vi "RGB to HSL.vi"(8 "error in (no error)":errorcluster, 9 "Blue":u8, 10 "Green":u8, 11 "Red":u8) -> (0 "error out":errorcluster, 1 "Lightness(%)":dbl format="%#_13g", 2 "Saturation(%)":dbl format="%#_13g", 3 "Hue(°)":dbl format="%#_13g")   [LabVIEW 2018]
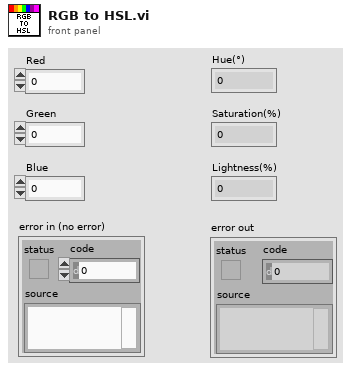
[diagram p1: front panel]
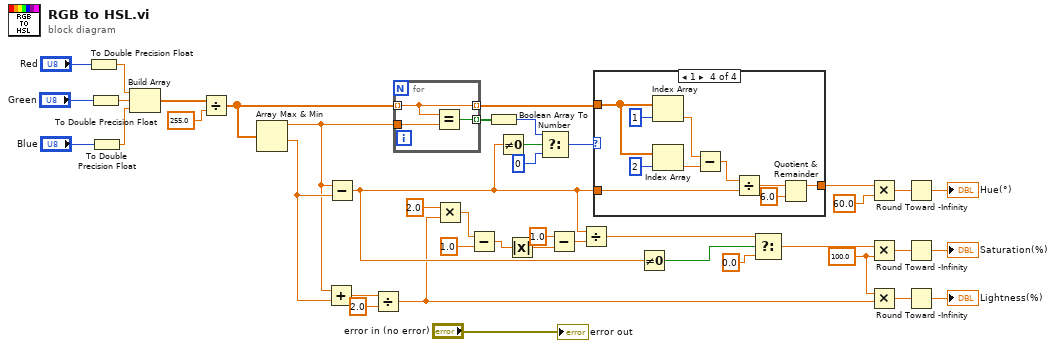
[diagram p0: block diagram]
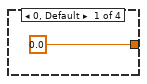
[diagram p2: hidden frame]
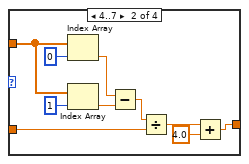
[diagram p3: hidden frame]
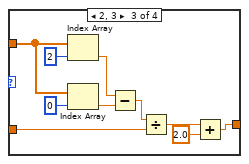
[diagram p4: hidden frame]
diagram:
  w31 = 100.0 ("x")
  n1 = To Double Precision Float(number="Red") -> (double precision float=w41:dbl)
  n2 = To Double Precision Float(number="Green") -> (double precision float=w40:dbl)
  n3 = To Double Precision Float(number="Blue") -> (double precision float=w39:dbl)
  n4 = Build Array(w41, w40, w39) -> (w38:dbl[])
  n5 = Divide(x=w38, y=255.0) -> (x/y=w20:dbl[])
  n6 = Array Max & Min(array=w20) -> (max value=w12:dbl, min value=w16:dbl)  [unwired: 2 out]
  n7 = Add(x=w12, y=w16) -> (x+y=w15:dbl)
  n8 = Subtract(x=w12, y=w16) -> (x-y=w19:dbl)
  n9 = Divide(x=w15, y=2.0) -> (x/y=w8:dbl)
  n10 = for {
    tunnel: w12 -> [w45]
    tunnel: [w44] -> w28 mode=indexing
    tunnel: w20 -> [w43] mode=indexing
    tunnel: [w43] -> w27 mode=indexing
    n11 = Equal?(x=w43, y=w45) -> (x = y?=w44:bool)
  }
  n12 = Multiply(x=2.0, y=w8) -> (x*y=w9:dbl)
  n13 = Subtract(x=w9, y=1.0) -> (x-y=w11:dbl)
  n14 = Boolean Array To Number(Boolean array=w28) -> (number=w24:u32)
  n15 = Not Equal To 0?(x=w19) -> (x != 0?=w25:bool)
  n16 = Absolute Value(x=w11) -> (abs(x)=w17:dbl)
  n17 = Select(t=w24, s=w25, f=u32 0) -> (s? t:f=w23:u32)
  n18 = Subtract(x=1.0, y=w17) -> (x-y=w13:dbl)
  n19 = Divide(x=w19, y=w13) -> (x/y=w35:dbl)
  n20 = case shown="1" w23 {
    tunnel: w27 -> [_ w49 w59 w72]
    tunnel: [0.0 ("x") w47 w57 w67] -> w26
    tunnel: w19 -> [_ w48 w58 w75]
    frame 0, Default {
    }
    frame 4..7 {
      n21 = Index Array(array=w49, index=0) -> (element=w52:dbl)
      n22 = Index Array(array=w49, index=1) -> (element=w51:dbl)
      n23 = Subtract(x=w52, y=w51) -> (x-y=w50:dbl)
      n24 = Divide(x=w50, y=w48) -> (x/y=w55:dbl)
      n25 = Add(x=w55, y=4.0) -> (x+y=w47:dbl)
    }
    frame 2, 3 {
      n26 = Index Array(array=w59, index=2) -> (element=w62:dbl)
      n27 = Index Array(array=w59, index=0) -> (element=w61:dbl)
      n28 = Subtract(x=w62, y=w61) -> (x-y=w60:dbl)
      n29 = Divide(x=w60, y=w58) -> (x/y=w65:dbl)
      n30 = Add(x=w65, y=2.0) -> (x+y=w57:dbl)
    }
    frame 1 {
      n31 = Index Array(array=w72, index=1) -> (element=w70:dbl)
      n32 = Index Array(array=w72, index=2) -> (element=w69:dbl)
      n33 = Subtract(x=w70, y=w69) -> (x-y=w68:dbl)
      n34 = Divide(x=w68, y=w75) -> (x/y=w74:dbl)
      n35 = Quotient & Remainder(x=w74, y=6.0) -> (x-y*floor(x/y)=w67:dbl)  [unwired: 1 out]
    }
  }
  n36 = Not Equal To 0?(x=w19) -> (x != 0?=w21:bool)
  n37 = Select(t=w35, s=w21, f=0.0 ("x")) -> (s? t:f=w33:dbl)
  n38 = Multiply(x=w26, y=60.0) -> (x*y=w30:dbl)
  n39 = Multiply(x=w33, y=w31) -> (x*y=w34:dbl)
  n40 = Multiply(x=w31, y=w8) -> (x*y=w32:dbl)
  n41 = Round Toward -Infinity(1:w30) -> (0:→"Hue(°)":dbl)
  n42 = Round Toward -Infinity(1:w34) -> (0:→"Saturation(%)":dbl)
  n43 = Round Toward -Infinity(1:w32) -> (0:→"Lightness(%)":dbl)
  "error out" <- "error in (no error)"
